vi "Parameters_Build_Stop.vi"(11 "Stop Mode":i32(ring)=11599968 items=["Decelerate"=11599968, "Immediate"=11599969, "Disable Drive"=11599970]) -> (3 "Parameters":dbl[](array[numeric]))   [LabVIEW 2017, in "WordManipulationLibrary.lvlib"]
uses:
  WordManipulationLibrary.lvlib
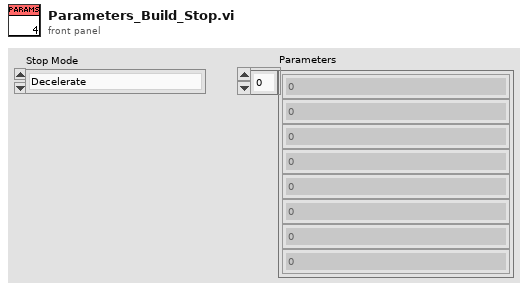
[diagram p1: front panel]
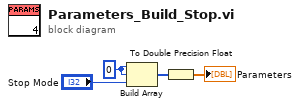
[diagram p0: block diagram]
diagram:
  w3 = 0 ("element")
  n1 = Build Array(w3, w3, "Stop Mode") -> (w1:i32[])
  n2 = To Double Precision Float(number=w1) -> (double precision float=→"Parameters":dbl[])
